vi "Get DAQ tasks.vi"(8 "error in":errorcluster, 9 "Camera":T1, 10 "Device Name":tag="Dev6", 11 "frequency":dbl=100.0 caption="Frecuencia PWM" format="%_6g") -> (0 "error out":errorcluster, 3 "Task list":T2)   [LabVIEW 2018]
uses:
  typedef/Task list.ctl
  <vilib>/vision/driver/NI_Vision_Acquisition_Software.lvlib
  <vilib>/DAQmx/write.llb/DAQmx Write (Digital 1D Bool 1Chan 1Samp).vi
  <vilib>/DAQmx/configure/timing.llb/DAQmx Timing (Implicit).vi
  <vilib>/DAQmx/create/channels.llb/DAQmx Create Channel (AI-Voltage-Basic).vi
  <vilib>/DAQmx/create/channels.llb/DAQmx Create Channel (CI-Position-Angular Encoder).vi
  <vilib>/DAQmx/create/channels.llb/DAQmx Create Channel (CO-Pulse Generation-Frequency).vi
  <vilib>/DAQmx/create/channels.llb/DAQmx Create Channel (DO-Digital Output).vi
  <vilib>/userDefined/High Color/IMAQdx.ctl
  <vilib>/vision/Image Controls.llb/IMAQ Image.ctl
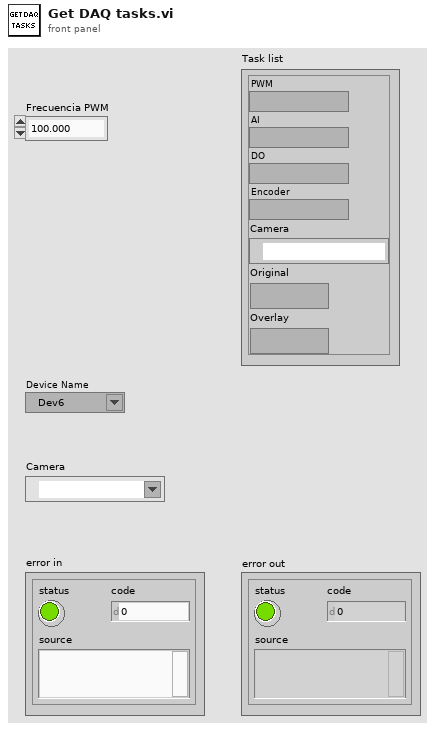
[diagram p1: front panel]
types:
  T1 = typedef "IMAQdx.ctl" = refnum<k21>
  T2 = typedef "Task list.ctl" = cluster{"PWM":refnum<k21>, "AI":refnum<k21>, "DO":refnum<k21>, "Encoder":refnum<k21>, "Camera":T1, "Original":T3, "Overlay":T3}
  T3 = typedef "IMAQ Image.ctl" = refnum<image>
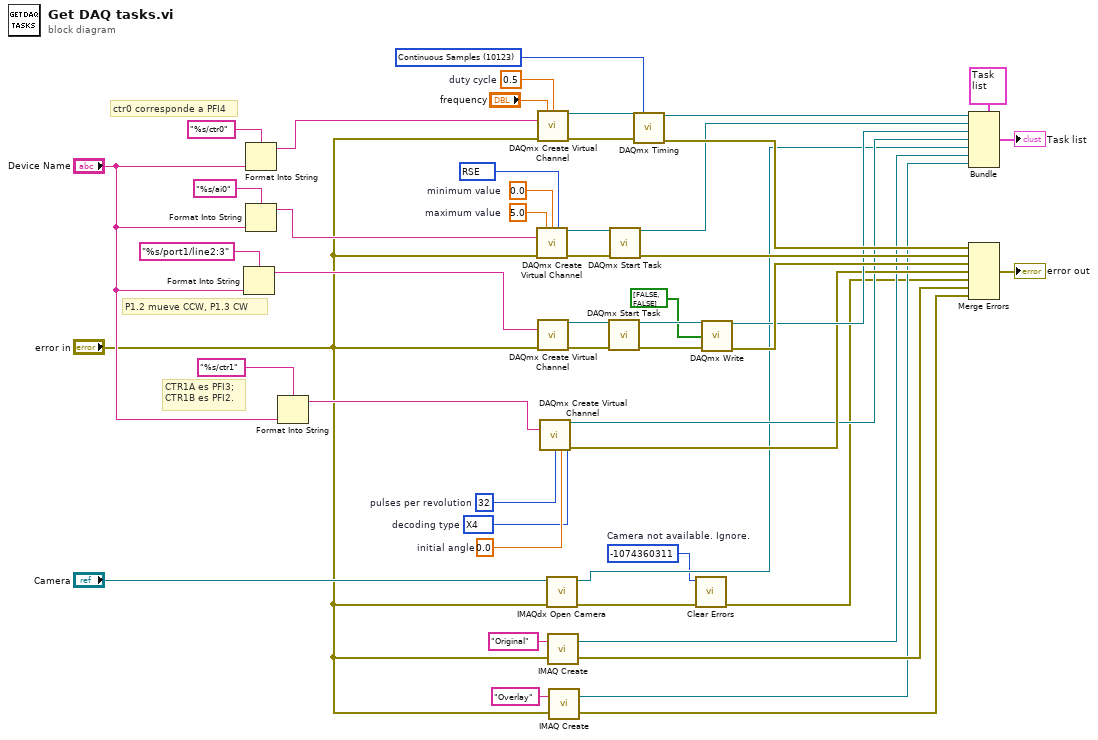
[diagram p0: block diagram]
diagram:
  w1 = -1074360311  # Camera not available. Ignore.
  w15 = 10092 items=["X1"=10090, "X2"=10091, "X4"=10092, "Two Pulse Counting"=10313]  # decoding type
  w16 = 0.0  # initial angle
  w17 = u32 32  # pulses per revolution
  w40 = 10083 items=["Default"=-1, "RSE"=10083, "NRSE"=10078, "Differential"=10106, "Pseudodifferential"=12529] ("input terminal configuration")
  w39 = 0.0  # minimum value
  w38 = 5.0  # maximum value
  w35 = 0.5  # duty cycle
  w31 = 10123 items=["Finite Samples"=10178, "Continuous Samples"=10123, "Hardware Timed Single Point"=12522] ("sample mode")
  # "CTR1A es PFI3;\nCTR1B es PFI2."
  # "P1.2 mueve CCW, P1.3 CW"
  # "ctr0 corresponde a PFI4"
  n1 = Format Into String(format string="%s/port1/line2:3", "Device Name") -> (resulting string=w50:string)  [unwired: 2 in, 1 out]
  n2 = Format Into String(format string="%s/ctr0", "Device Name") -> (resulting string=w48:string)  [unwired: 2 in, 1 out]
  n3 = Format Into String(format string="%s/ai0", "Device Name") -> (resulting string=w49:string)  [unwired: 2 in, 1 out]
  n4 = Format Into String(format string="%s/ctr1", "Device Name") -> (resulting string=w18:string)  [unwired: 2 in, 1 out]
  n5 = call-poly <vilib>:"DAQmx Create Virtual Channel.vi"("maximum value"=w38, "minimum value"=w39, "input terminal configuration"=w40, "physical channels"=w49, "error in"="error in") -> ("task out"=w43:refnum<k21>, "error out"=w42:errorcluster)  [unwired: 9 in]
  n6 = call-poly <vilib>:"DAQmx Create Virtual Channel.vi"("frequency"="frequency", "duty cycle"=w35, "counter"=w48, "error in"="error in") -> ("task out"=w33:refnum<k21>, "error out"=w32:errorcluster)  [unwired: 10 in]
  n7 = call-poly <vilib>:"DAQmx Create Virtual Channel.vi"("lines"=w50, "error in"="error in") -> ("task out"=w37:refnum<k21>, "error out"=w36:errorcluster)  [unwired: 12 in]
  n8 = call-poly <vilib>:"DAQmx Create Virtual Channel.vi"("counter"=w18, "decoding type"=w15, "pulses per revolution"=w17, "initial angle"=w16) -> ("task out"=w13:refnum<k21>, "error out"=w14:errorcluster)  [unwired: 10 in]
  n9 = call <vilib>:"IMAQdx Open Camera.vi"("error in"="error in", "Session In"="Camera") -> ("error out"=w11:errorcluster, "Session Out"=w10:T1)  [unwired: 8 in]
  n10 = call "IMAQ Create"("Image Name"="Original", "error in (no error)"="error in") -> ("New Image"=w4:T3, "error out"=w6:errorcluster)  [unwired: 3 in]
  n11 = call "IMAQ Create"("Image Name"="Overlay", "error in (no error)"="error in") -> ("New Image"=w3:T3, "error out"=w5:errorcluster)  [unwired: 3 in]
  n12 = call <vilib>:"DAQmx Start Task.vi"("task/channels in"=w37, "error in"=w36) -> ("task out"=w23:refnum<k21>, "error out"=w41:errorcluster)  [unwired: 12 in]
  n13 = call <vilib>:"DAQmx Start Task.vi"("task/channels in"=w43, "error in"=w42) -> ("task out"=w29:refnum<k21>, "error out"=w44:errorcluster)  [unwired: 12 in]
  n14 = call-poly <vilib>:"DAQmx Timing.vi"("task/channels in"=w33, "sample mode"=w31, "error in"=w32) -> ("task out"=w30:refnum<k21>, "error out"=w45:errorcluster)  [unwired: 11 in]
  n15 = call <vilib>:"Clear Errors.vi"("error in (no error)"=w11, "specific error code to clear (0: all)"=w1) -> ("error out"=w2:errorcluster)  [unwired: 4 in, 1 out]
  n16 = call-poly <vilib>:"DAQmx Write.vi"("task/channels in"=w23, "data"=bool[] [FALSE, FALSE], "error in"=w41) -> ("task out"=w22:refnum<k21>, "error out"=w24:errorcluster)  [unwired: 10 in, 1 out]
  n17 = Bundle(cluster=T2 {"PWM"="", "AI"="", "DO"="", "Encoder"="", "Camera"="", "Original"=refnum, "Overlay"=refnum} ("Task list"), "PWM"=w30, "AI"=w29, "DO"=w22, "Encoder"=w13, "Camera"=w10, "Original"=w4, "Overlay"=w3) -> (→"Task list":T2)
  n18 = Merge Errors(w45, w44, w24, w14, w2, w6, w5) -> (→"error out":errorcluster)
